vi "P12.vi"() -> ()   [LabVIEW 2018]
uses:
  <vilib>/vision/NI_Vision_Development_Module.lvlib
panel:
  out "error out":errorcluster
  out "Waveform Graph":cluster{"x0":sgl, "dx":sgl, "Pixels Line":sgl[]}(graph)
  in  "stop":bool
  in  "error in (no error)":errorcluster
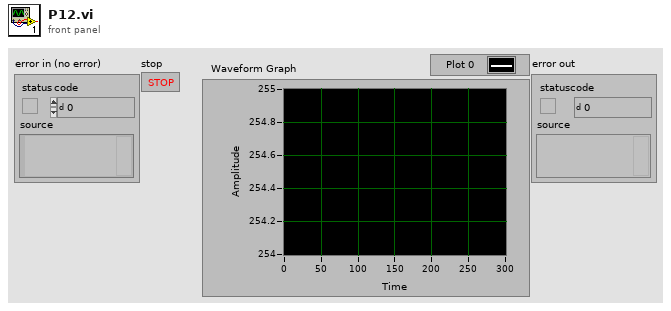
[diagram p1: front panel]
types:
  T1 = typedef "Image Type" = u32
  T2 = typedef "IMAQ Image.ctl" = refnum<image>
  T3 = typedef "ROI Descriptor" = cluster{"Global Rectangle":i32[], "Contours":cluster{"ID":enum32{"External", "Internal"}, "Type":u32, "Coordinates":i32[]}[]}
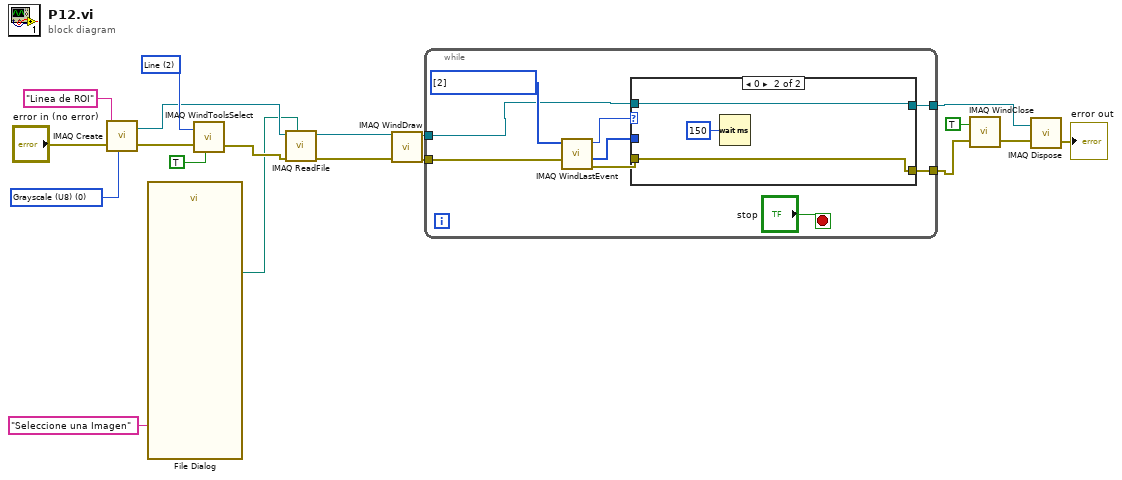
[diagram p0: block diagram]
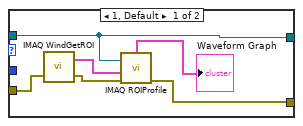
[diagram p2: hidden frame]
diagram:
  w15 = u32 2 items=["No Selection", "Point", "Line", "Rectangle", "Oval", "Polygon", "Freehand Region", "Annulus", "Zoom", "Pan", "Broken Line", "Freehand Line", "Rotated Rectangle"] ("Tool (Point)")
  w17 = T1 0 items=["Grayscale (U8)", "Grayscale (I16)", "Grayscale (SGL)", "Complex (CSG)", "RGB (U32)", "HSL (U32)", "RGB (U64)", "Grayscale (U16)"] ("Image Type")
  n1 = call "IMAQ Create"("Image Name"="Linea de ROI", "Image Type"=w17, "error in (no error)"="error in (no error)") -> ("New Image"=w14:T2, "error out"=w16:errorcluster)  [unwired: 2 in]
  n2 = call "File Dialog"("prompt"="Seleccione una Imagen") -> ("selected path"=w10:path)  [unwired: 11 in, 3 out]
  n3 = call "IMAQ WindToolsSelect"("Tool (Point)"=w15, "Get/Set Status? (Set)"=TRUE, "error in (no error)"=w16) -> ("error out"=w13:errorcluster)  [unwired: 2 in, 1 out]
  n4 = call <userlib>:"IMAQ ReadFile.vi"("File Path"=w10, "error in (no error)"=w13, "Image"=w14) -> ("error out"=w9:errorcluster, "Image Out"=w8:T2)  [unwired: 4 in, 3 out]
  n5 = call "IMAQ WindDraw"("error in (no error)"=w9, "Image"=w8) -> ("error out"=w6:errorcluster, "Image Out (duplicate)"=w7:T2)  [unwired: 8 in]
  n6 = while {
    tunnel: w7 -> [w25]
    tunnel: w6 -> [w27]
    tunnel: [w21] -> w2
    tunnel: [w20] -> w3
    stop <- "stop" stop-if-true
    w26 = i32[] [2] items=["No  event", "Click event", "Draw event", "Move event", "Size event", "Scroll event", "Activate event", "Close event", "Double click event"] ("Events list (all)")
    n7 = call "IMAQ WindLastEvent"("error in (no error)"=w27, "Events list (all)"=w26) -> ("error out"=w23:errorcluster, "Coordinates"=w22:i32[], "Event"=w24:i32)  [unwired: 4 in, 3 out]
    n8 = case shown="0" w24 {
      tunnel: w25 -> [w31 w37]
      tunnel: w23 -> [w34 w36]
      tunnel: w22 -> [_ _]
      tunnel: [w31 w37] -> w21
      tunnel: [w29 w36] -> w20
      frame 1, Default {
        n9 = call "IMAQ WindGetROI"("error in (no error)"=w34) -> ("ROI Descriptor"=w33:T3, "error out"=w32:errorcluster)  [unwired: 4 in]
        n10 = call "IMAQ ROIProfile"("error in (no error)"=w32, "ROI Descriptor"=w33, "Image"=w31) -> ("error out"=w29:errorcluster, "ROI Graph"=→"Waveform Graph":cluster{"x0":sgl, "dx":sgl, "Pixels Line":sgl[]})  [unwired: 1 in, 3 out]
      }
      frame 0 {
        n11 = Wait (ms)(milliseconds to wait=u32 150) -> ()  [unwired: 1 out]
      }
    }
  }
  n12 = call "IMAQ WindClose"("Close All Windows (False)"=TRUE, "error in (no error)"=w3) -> ("error out"=w5:errorcluster)  [unwired: 4 in]
  n13 = call "IMAQ Dispose"("Image"=w2, "error in (no error)"=w5) -> ("error out"=→"error out":errorcluster)  [unwired: 4 in]
